vi "createImageRefnum.vi"(8 "error in":errorcluster, 11 "Output cluster in":T1) -> (0 "error out":errorcluster, 3 "Output cluster out":T1)   [LabVIEW 2020]
doc: "Create refnum from image object"
uses:
  controls/StateMachineVariables.ctl
  <vilib>/vision/Avi.llb/IMAQ AVI2 Refnum.ctl
  <vilib>/userDefined/High Color/IMAQdx.ctl
  <vilib>/vision/Deep Learning.llb/IMAQ DL Model Refnum.ctl
  <vilib>/vision/Image Controls.llb/IMAQ Image.ctl
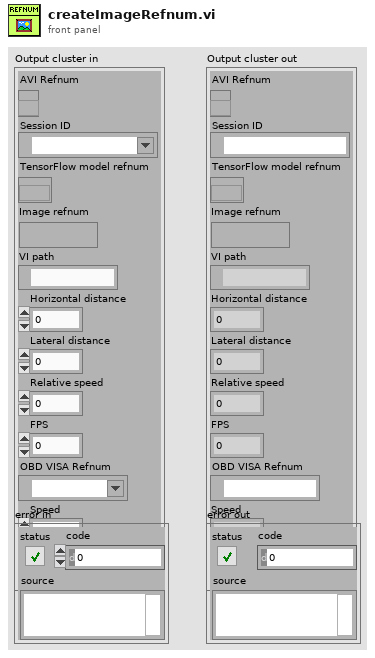
[diagram p1: front panel]
types:
  T1 = typedef "StateMachineVariables.ctl" = cluster{"AVI Refnum":T2, "Session ID":T3, "TensorFlow model refnum":T4, "Image refnum":T5, "VI path":path, "Horizontal distance":dbl, "Lateral distance":dbl, "Relative speed":dbl, "FPS":dbl, "OBD VISA Refnum":refnum<visa-resource-name>, "Speed":dbl, "Frame multiplier":u32}
  T2 = typedef "IMAQ AVI2 Refnum.ctl" = refnum<k20>
  T3 = typedef "IMAQdx.ctl" = refnum<k21>
  T4 = typedef "IMAQ DL Model Refnum.ctl" = refnum<k20>
  T5 = typedef "IMAQ Image.ctl" = refnum<image>
  T6 = typedef "Image Type" = u32
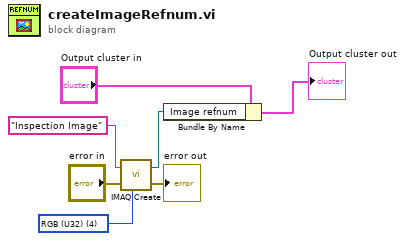
[diagram p0: block diagram]
diagram:
  w4 = T6 4 items=["Grayscale (U8)", "Grayscale (I16)", "Grayscale (SGL)", "Complex (CSG)", "RGB (U32)", "HSL (U32)", "RGB (U64)", "Grayscale (U16)"] ("Image Type")
  n1 = call "IMAQ Create"("Image Name"="Inspection Image", "Image Type"=w4, "error in (no error)"="error in") -> ("New Image"=w5:T5, "error out"=→"error out":errorcluster)  [unwired: 2 in]
  n2 = Bundle By Name(cluster="Output cluster in", "Image refnum"=w5) -> (→"Output cluster out":T1)
